vi "MAIN_change_image_orientation.vi"(3 "error in":errorcluster, 5 "Image IN":T1) -> (0 "error out":errorcluster, 2 "Image Out":T1)   [LabVIEW 2015]
uses:
  <vilib>/vision/Image Controls.llb/IMAQ Image.ctl
  <vilib>/vision/NI_Vision_Development_Module.lvlib
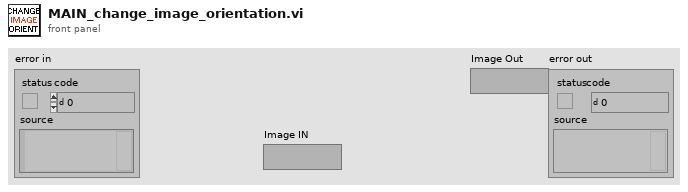
[diagram p1: front panel]
types:
  T1 = typedef "IMAQ Image.ctl" = refnum<image>
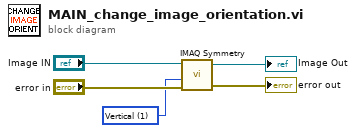
[diagram p0: block diagram]
diagram:
  w1 = u32 1 items=["Horizontal", "Vertical", "Central", "1st Diagonal", "2nd Diagonal"] ("Type of Symmetry")
  n1 = call "IMAQ Symmetry"("error in (no error)"="error in", "Type of Symmetry"=w1, "Image Src"="Image IN") -> ("error out"=→"error out":errorcluster, "Image Dst Out"=→"Image Out":T1)  [unwired: 2 in]
